vi "Load Notebook Themes.vi"(8 "error in":errorcluster) -> (0 "error out":errorcluster, 1 "# Loaded Themes":i32, 3 "File Path":path, 4 "Message":string)   [LabVIEW 2021, in "Notebook.lvlib"]
uses:
  Notebook.lvlib
  Notebook Parameters List.ctl
  Notebook Theme.ctl
  Rich Text Box/Named Text Style.ctl
  Rich Text Box/Text Formatting.ctl
  Rich Text Box/Text Colors.ctl
  Rich Text Box/Text Style.ctl
  Rich Text Box/Text Alignment.ctl
  0da9f478-be9e-4823-a999-d404b94a1446.vi
  <vilib>/JDP Science/JSONtext/JSON text to Variant.vi
  <vilib>/JDP Science/JSONtext/LVClass Serializer/JSONtext LVClass Serializer.lvclass
  Rich Text Box/Rich Text Box.lvlib
panel:
  # "see the License on the block diagram (Ctrl+E or Window:Show Block Diagram)"
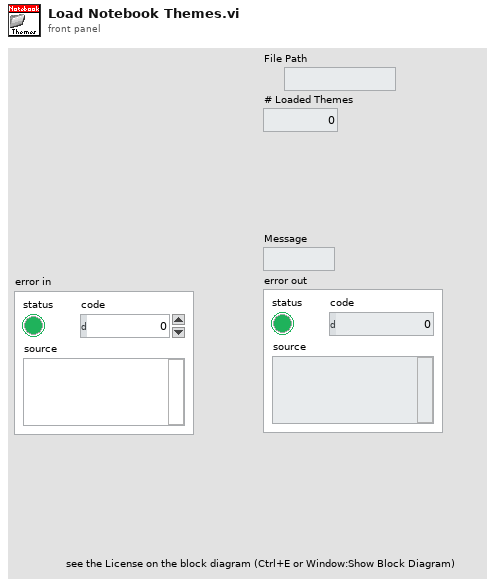
[diagram p1: front panel]
types:
  T1 = typedef "Notebook.lvlib/Notebook Theme.ctl" = cluster{"Theme Name":string, "[Named Text Styles]":T2[], "Page Color":T4}
  T2 = typedef "Notebook.lvlib/Named Text Style.ctl" = cluster{"Text Formatting":T3, "Text Style Name":string}
  T3 = typedef "Rich Text Box.lvlib/Text Formatting.ctl" = cluster{"Font":string, "Text Color":T4, "Background Color":T4, "Style":T5, "Font Size":dbl, "Alignment":T6}
  T4 = typedef "Rich Text Box.lvlib/Text Colors.ctl" = enum16{"Unchanged", "Black", "Blue", "Cyan", "Maroon", "Gray", "Violet", "Green", "Light Green", "Orange", "Yellow", "Magenta", "Red", "White"}
  T5 = typedef "Rich Text Box.lvlib/Text Style.ctl" = enum16{"Regular", "Bold", "Italic", "Underline", "Strikeout"}
  T6 = typedef "Rich Text Box.lvlib/Text Alignment.ctl" = enum16{"Left", "Right", "Center"}
  T7 = typedef "Notebook.lvlib/Notebook Parameters List.ctl" = enum16{"First Opening?", "Saved Notebook?", "Saved Notebook Path", "Beep on Error?", "Notebook Themes", "Current Theme Name"}
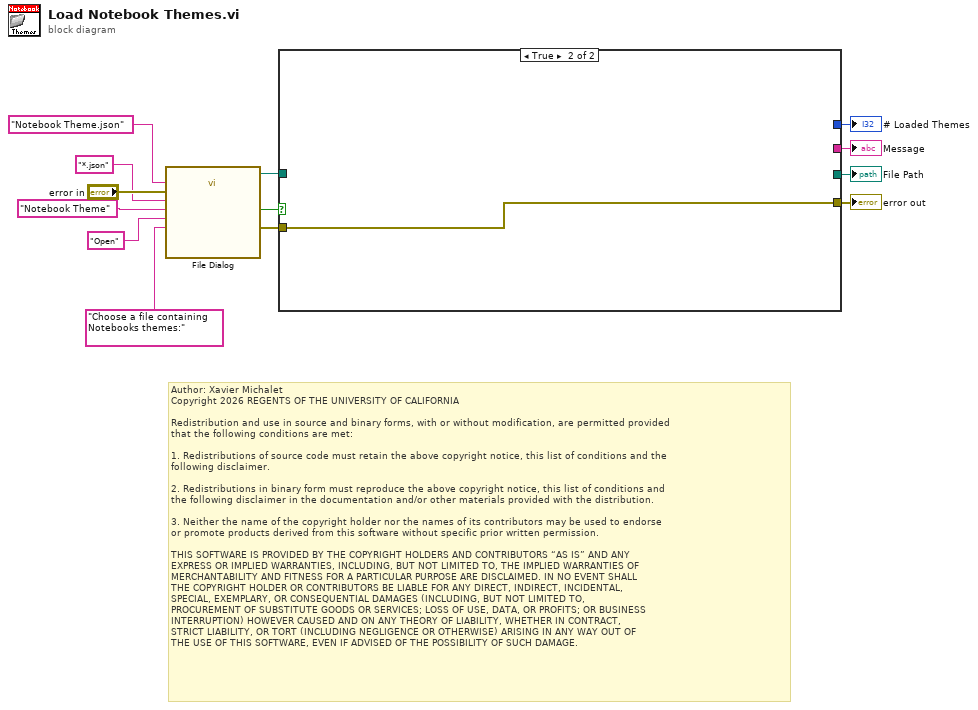
[diagram p0: block diagram]
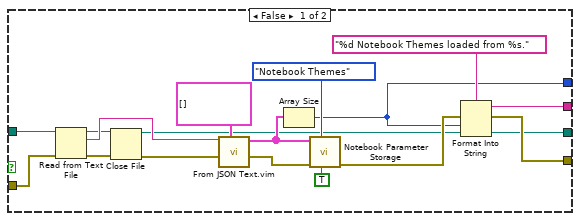
[diagram p2: hidden frame]
diagram:
  # "Author: Xavier Michalet\nCopyright 2026 REGENTS OF THE UNIVERSITY OF CALIFORNIA\n\nRedistribution and use in source and binary forms, with or without modification, are permitted provided\nthat the following conditions are met:\n\n1. Redistributions of source code must retain the above copyright notice, this list of conditions and the\nfollowing disclaimer.\n\n2. Redistributions in binary form must reproduce the above copyright notice, this list of conditions and\nthe following disclaimer in the documentation and/or other materials provided with the distribution.\n\n3. Neither the name of the copyright holder nor the names of its contributors may be used to endorse \nor promote products derived from this software without specific prior written permission.\n\nTHIS SOFTWARE IS PROVIDED BY THE COPYRIGHT HOLDERS AND CONTRIBUTORS “AS IS” AND ANY \nEXPRESS OR IMPLIED WARRANTIES, INCLUDING, BUT NOT LIMITED TO, THE IMPLIED WARRANTIES OF\nMERCHANTABILITY AND FITNESS FOR A PARTICULAR PURPOSE ARE DISCLAIMED. IN NO EVENT SHALL\nTHE COPYRIGHT HOLDER OR CONTRIBUTORS BE LIABLE FOR ANY DIRECT, INDIRECT, INCIDENTAL, \nSPECIAL, EXEMPLARY, OR CONSEQUENTIAL DAMAGES (INCLUDING, BUT NOT LIMITED TO, \nPROCUREMENT OF SUBSTITUTE GOODS OR SERVICES; LOSS OF USE, DATA, OR PROFITS; OR BUSINESS\nINTERRUPTION) HOWEVER CAUSED AND ON ANY THEORY OF LIABILITY, WHETHER IN CONTRACT, \nSTRICT LIABILITY, OR TORT (INCLUDING NEGLIGENCE OR OTHERWISE) ARISING IN ANY WAY OUT OF\nTHE USE OF THIS SOFTWARE, EVEN IF ADVISED OF THE POSSIBILITY OF SUCH DAMAGE."
  n1 = call "File Dialog"("prompt"="Choose a file containing Notebooks themes:" ("prompt (Choose or enter file path)"), "button label"="Open", "default name"="Notebook Theme.json", "error in"="error in", "pattern (all files)"="*.json", "pattern label"="Notebook Theme") -> ("selected path"=w13:path, "cancelled"=w11:bool, "error out"=w12:errorcluster)  [unwired: 6 in, 1 out]
  n2 = case shown="True" w11 {
    tunnel: w13 -> [w19 _]
    tunnel: w12 -> [w18 w31]
    tunnel: [w17 _] -> w10
    tunnel: [w16 w31] -> w9
    tunnel: [w15 _] -> w8
    tunnel: [w14 _] -> w7
    frame False {
      n3 = Read from Text File(file (use dialog)=w19, error in=w18) -> (refnum out=w22:refnum<file>, text=w25:string, error out=w23:errorcluster)  [unwired: 2 in, 1 out]
      n4 = Close File(refnum=w22, error in=w23) -> (path=w15:path, error out=w24:errorcluster)
      n5 = call "From JSON Text.vim"("Data Type and Default Value"=T1[] [] ("Array"), "error in (no error)"=w24, "JSON"=w25) -> ("error out"=w27:errorcluster, "Data out"=w29:T1[])  [unwired: 7 in]
      n6 = Array Size(array=w29) -> (size(s)=w14:i32)
      n7 = call "Notebook Parameter Storage.vi"("Get(F)/Set"=TRUE, "Notebook Parameter List"=Notebook_Parameters_List."Notebook Themes", "Error In"=w27, "Data in"=w29) -> ("Error Out"=w30:errorcluster)  [unwired: 6 in, 1 out]
      n8 = Format Into String(format string="%d Notebook Themes loaded from %s.", error in=w30, w14, w15) -> (resulting string=w17:string, error out=w16:errorcluster)  [unwired: 1 in]
    }
    frame True {
    }
  }
  "Message" <- w10
  "error out" <- w9
  "File Path" <- w8
  "# Loaded Themes" <- w7
